vi "Move Window.vi"(8 "error in":errorcluster caption="error in (no error)" {"code" format="%d\n%x"}, 9 "new position (0,0)":cluster{"left":i16, "top":i16}, 10 "window name (\"\")":string, 11 "window refnum":T1 caption="window refnum (NaWR)") -> (0 "error out":errorcluster {"code" format="%d\n%x"}, 1 "prev position":cluster{"left":i16, "top":i16}, 3 "window refnum out":T1)   [LabVIEW 2020, in "MacroAssert.lvlib" / "Win Util New.lvlib"]
doc: "This function will move the window named in the 'window name' input or identified by the 'window refnum' from its present location to that defined in the 'new position' cluster. Coordinates are pixels relative to upper left corner of the screen.\n\nIf the function is successful, then:\n'window refnum out' = 'window refnum' if window refnum in is valid;\n'window refnum out' is a new window refnum if 'window refnum' is not valid and 'window name' a valid name for a window.\n\nIf the window cannot be found, an error will be returned and window refnum out will be 'Not a Valid Window RefNum'."
uses:
  Win Util New.lvlib
  Window Refnum.ctl
  user32.dll
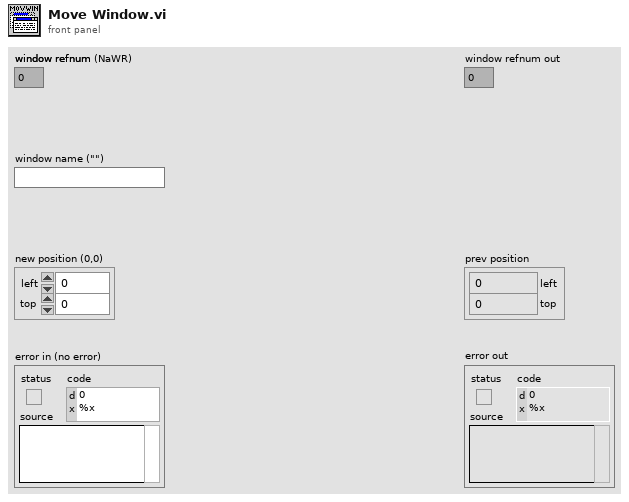
[diagram p1: front panel]
types:
  T1 = typedef "MacroAssert.lvlib/Win Util New.lvlib/Window Refnum.ctl" = u64
  T2 = cluster{"left":i16, "top":i16, "right":i16, "bottom":i16}
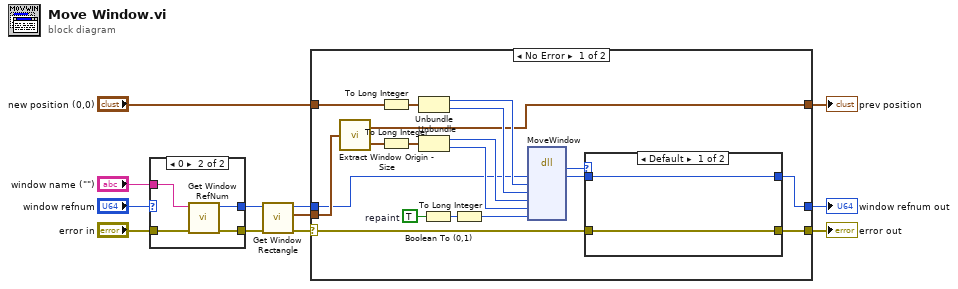
[diagram p0: block diagram]
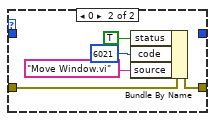
[diagram p3: hidden frame]
diagram:
  n1 = case shown="0" "window refnum" {
    selector: "window refnum" -> [w13 _]
    tunnel: "error in" -> [w14 w18]
    tunnel: [w13 w17] -> w7
    tunnel: [w14 w16] -> w8
    tunnel: "window name (\"\")" -> [_ w15]
    frame Default {
    }
    frame 0 {
      n2 = call "Get Window RefNum.vi"("error in"=w18, "window name (\"\")"=w15) -> ("error out"=w16:errorcluster, "window refnum (NaWR)"=w17:T1)  [unwired: 6 out]
    }
  }
  n3 = call "Get Window Rectangle.vi"("error in"=w8, "window refnum (NaWR)"=w7) -> ("error out"=w3:errorcluster, "window rect"=w10:T2, "window refnum out"=w11:T1)  [unwired: 7 in]
  n4 = case shown="No Error" w3 {
    selector: w3 -> [w27 w46]
    tunnel: w10 -> [w31 _]
    tunnel: [w30 w46] -> w12
    tunnel: w11 -> [w28 w47]
    tunnel: [w24 w47] -> w9
    tunnel: "new position (0,0)" -> [w29 w45]
    tunnel: [w23 w45] -> w1
    frame No Error {
      w34 = TRUE  # repaint
      n5 = call "Extract Window Origin - Size.vi"("window rect"=w31) -> ("window origin"=w23:cluster{"left":i16, "top":i16}, "window size"=w35:cluster{"Width":i16, "Height":i16})
      n6 = To Long Integer(number=w29) -> (32bit integer=w21:cluster{"left":i32, "top":i32})
      n7 = To Long Integer(number=w35) -> (32bit integer=w20:cluster{"Width":i32, "Height":i32})
      n8 = Unbundle(w21) -> ("left"=w37:i32, "top"=w36:i32)
      n9 = Unbundle(w20) -> ("Width"=w33:i32, "Height"=w32:i32)
      n10 = Boolean To (0,1)(Boolean=w34) -> (0, 1=w22:i16)
      n11 = To Long Integer(number=w22) -> (32bit integer=w19:i32)
      n12 = dll-call lib="USER32.DLL" fn="MoveWindow"("hWnd"=w28, "left"=w37, "top"=w36, "right"=w33, "bottom"=w32, "repaint"=w19) -> ("error"=w26:i32, "hWnd"=w25:u64)  [unwired: 3 in, 7 out]
      n13 = case shown="Default" w26 {
        tunnel: [w39 w44] -> w30
        tunnel: w27 -> [w39 w43]
        tunnel: w25 -> [w38 _]
        tunnel: [w38 _] -> w24
        frame Default {
        }
        frame 0 {
          n14 = Bundle By Name(cluster=w43, "status"=TRUE, "code"=6021, "source"="Move Window.vi") -> (w44:errorcluster)
        }
      }
    }
    frame Error {
    }
  }
  "error out" <- w12
  "window refnum out" <- w9
  "prev position" <- w1
